vi "Test wrapper.vi"() -> ()   [LabVIEW 2009]
uses:
  <vilib>/Analysis/2dsp.llb/2D Complex FFT.vi
  <vilib>/Analysis/NI_AALPro.lvlib
panel:
  in  "Save\nAmplitudes":bool
  in  "deviceId":i32
  in  "Intensity":sgl[](array[numeric])=[1.0, 1.0, 1.0]
  in  "Polynomial Coefficients":sgl[](array[numeric])=[128.0, 0.0, 0.0, 40.0, 0.0, 0.0, 0.0, 0.0, 0.0, 0.0, 0.0, 0.0, 0.0, 0.0, 0.0, 0.0, 0.0, 0.0, 0.0, 0.0, 0.0, 0.0, 0.0, 0.0, 0.0, 0.0, 0.0, 0.0, 0.0, 0.0, 0.0, 0.0, 0.0, 0.0, 0.0, 0.0, 0.0, 0.0, 0.0, 0.0, 0.0, 0.0, 0.0, 0.0, 0.0, 0.0, 0.0, 0.0, 0.0, 0.0, 0.0, 0.0, 0.0, 0.0, 0.0, 0.0, 0.0, 0.0, 0.0, 0.0, 0.0, 0.0, 0.0, 0.0, 0.0, 0.0, 0.0, 0.0, 0.0, 0.0, 0.0, 0.0, 0.0, 0.0, 0.0, 0.0, 0.0, 0.0, 0.0, 0.0, 0.0, 0.0, 0.0, 0.0, 0.0, 0.0, 0.0, 0.0, 0.0, 0.0, 0.0, 0.0, 0.0, 0.0, 0.0, 0.0, 0.0, 0.0, 0.0, 0.0, 0.0, 0.0, 0.0, 0.0, 0.0, 0.0, 0.0, 0.0, 0.0, 0.0, 0.0, 0.0, 0.0, 0.0, 0.0, 0.0, 0.0, 0.0, 0.0, 0.0]
  in  "alpha RPC":sgl=1.0
  in  "Polynomial Order":i32=3 min=3 max=7 step=1
  in  "Use polynomial LUT":bool=TRUE
  out "error out":errorcluster
  in  "Aberration Correction On":bool
  in  "Aberration Correction":sgl[](array[numeric])=array[262144 elements]
  in  "TrueFrame":i32=3
  in  "Number of \ntime to execute":i32=1
  out "Average \nexecution time":dbl=nan
  in  "GO":bool
  in  "stop program":bool
  out "Amplitudes/weights":sgl[][](graph)=[[1.0001239, 1.0001477, 1.0001446, 1.0001416, 1.0001386, 1.0001358, 1.0001332, 1.0001305, 1.0001283, 1.0001258], [0.99984175, 0.99979293, 0.9997994, 0.99980545, 0.9998114, 0.9998169, 0.9998223, 0.99982744, 0.9998326, 0.9998372], [1.0000381, 1.0000628, 1.0000595, 1.0000563, 1.0000532, 1.0000505, 1.0000477, 1.0000453, 1.0000426, 1.0000404]]
  out "Calculated image plane":dbl[][](graph)
  out "Generated Hologram":u8[][](graph)
  in  "method":i32(ring)=1 items=["Lenses and Gratings (3D)", "Gerchberg-Saxton (3D)", "Gerchberg-Saxton FFT (2D)"]
  in  "z":sgl[](array[numeric])=[0.0, 0.0, 0.0]
  in  "y":sgl[](array[numeric])=[4.0, 5.0, -4.0]
  in  "x":sgl[](array[numeric])=[4.0, -4.0, 4.0]
  in  "N_iterations":i32=10
  in  "SLM enabled":bool
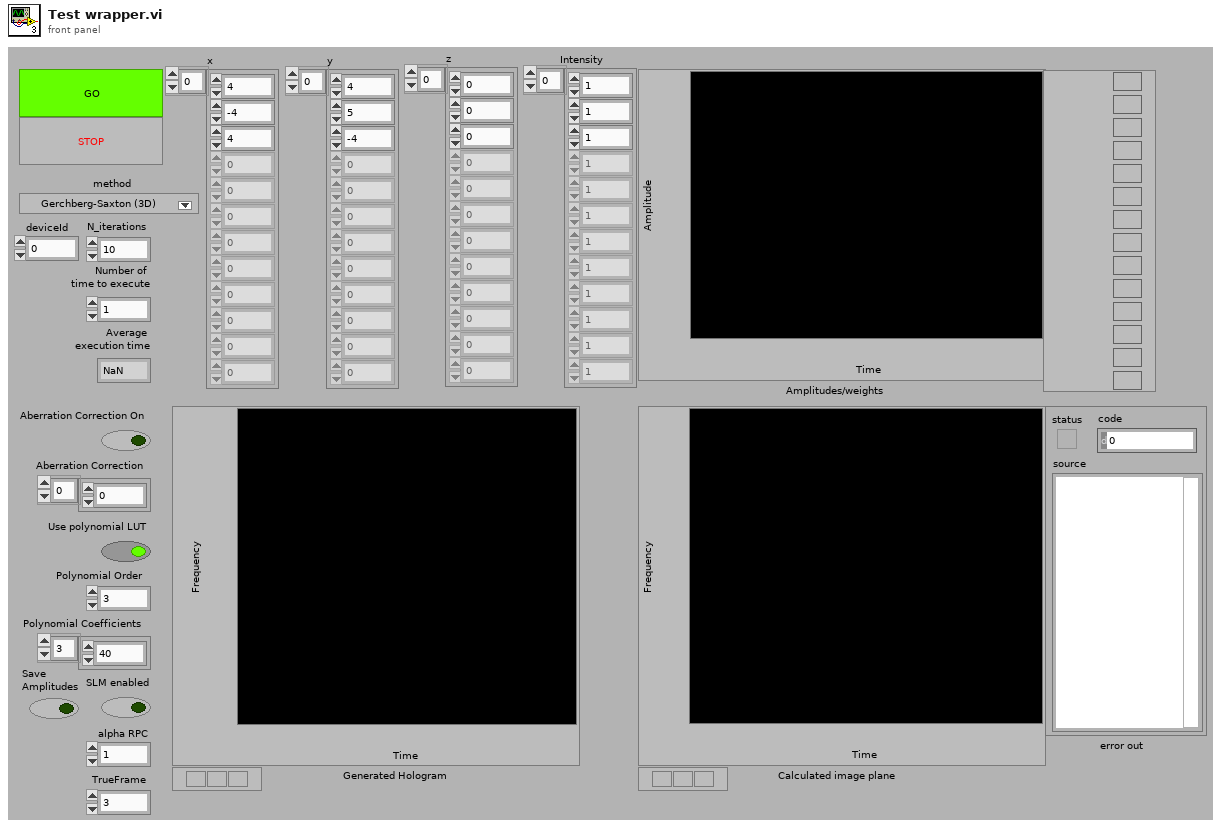
[diagram p1: front panel]
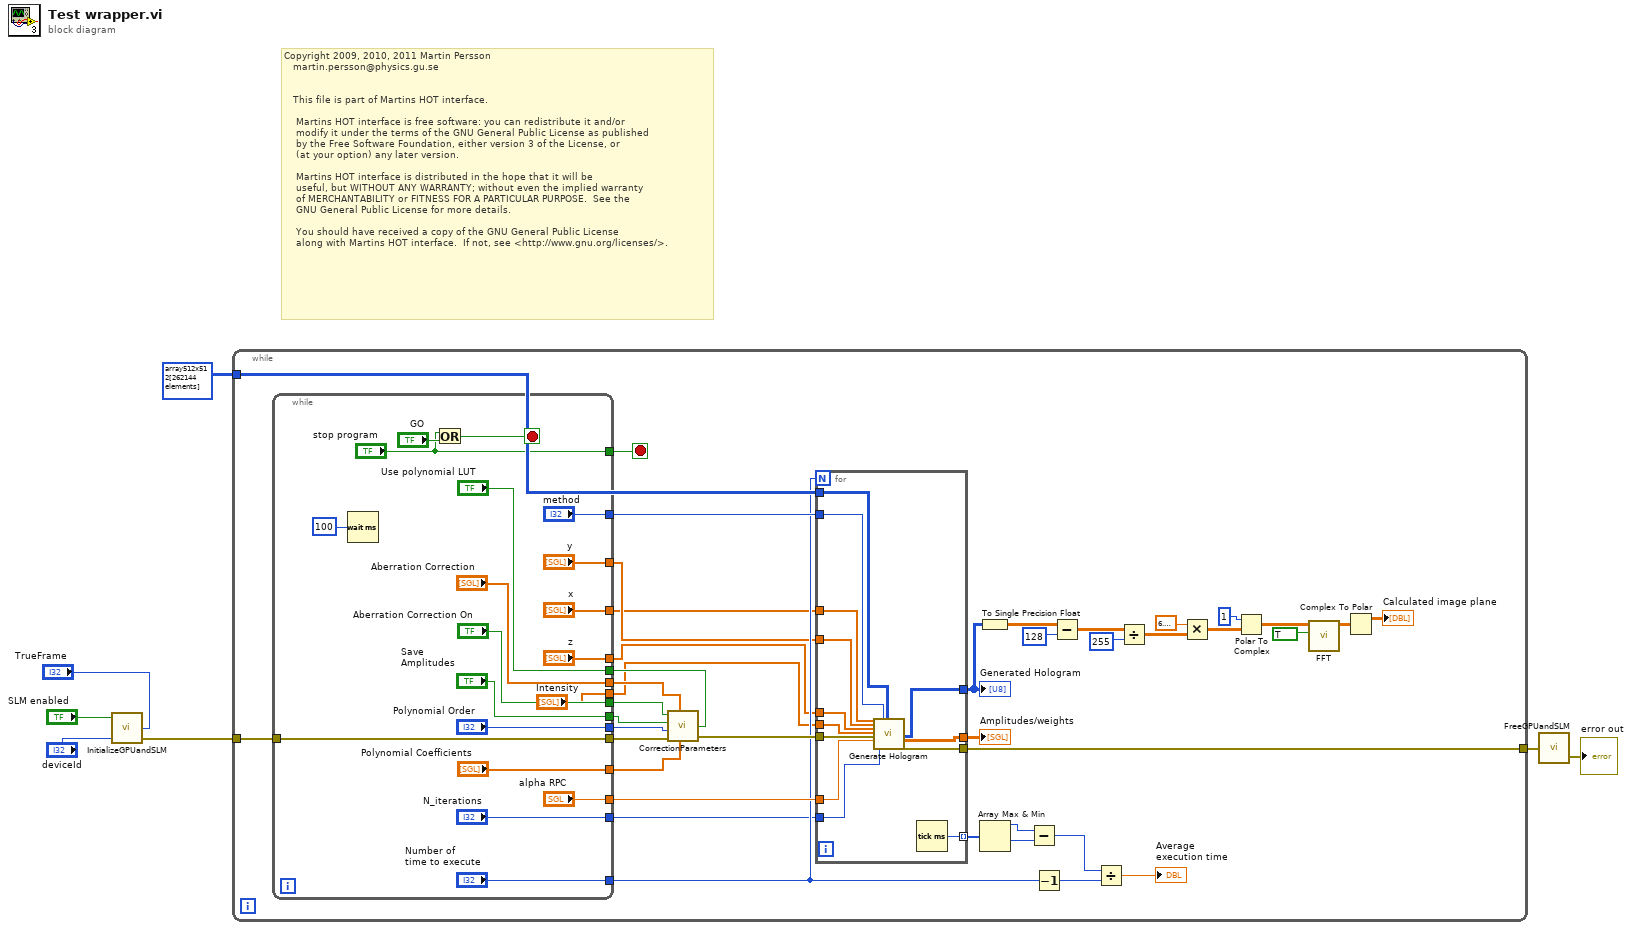
[diagram p0: block diagram]
diagram:
  # "Copyright 2009, 2010, 2011 Martin Persson \n   martin.persson@physics.gu.se\n\n\n   This file is part of Martins HOT interface.\n\n    Martins HOT interface is free software: you can redistribute it and/or \n    modify it under the terms of the GNU General Public License as published \n    by the Free Software Foundation, either version 3 of the License, or\n    (at your option) any later version.\n\n    Martins HOT interface is distributed in the hope that it will be \n    useful, but WITHOUT ANY WARRANTY; without even the implied warranty\n    of MERCHANTABILITY or FITNESS FOR A PARTICULAR PURPOSE.  See the\n    GNU General Public License for more details.\n\n    You should have received a copy of the GNU General Public License\n    along with Martins HOT interface.  If not, see <http://www.gnu.org/licenses/>."
  n1 = call "InitializeGPUandSLM.vi"("TrueFrame"="TrueFrame", "deviceId"="deviceId", "SLM enabled"="SLM enabled") -> ("CUDA/SLM error"=w1:errorcluster)  [unwired: 1 in, 1 out]
  n2 = while {
    tunnel: w1 -> [w24]
    tunnel: [w45] -> w6
    tunnel: u8[][] array512x512[262144 elements] ("Default") -> [w32]
    stop <- w46 stop-if-true
    n3 = while {
      tunnel: ["stop program"] -> w46
      tunnel: w24 -> [w75]
      tunnel: [w75] -> w23
      tunnel: ["alpha RPC"] -> w21
      tunnel: ["Use polynomial LUT"] -> w20
      tunnel: ["Aberration Correction On"] -> w19
      tunnel: ["method"] -> w18
      tunnel: ["Number of \ntime to execute"] -> w17
      tunnel: ["y"] -> w16
      tunnel: ["z"] -> w15
      tunnel: ["x"] -> w14
      tunnel: ["Polynomial Order"] -> w13
      tunnel: ["Aberration Correction"] -> w12
      tunnel: ["Polynomial Coefficients"] -> w11
      tunnel: ["N_iterations"] -> w10
      tunnel: ["Intensity"] -> w9
      tunnel: ["Save\nAmplitudes"] -> w8
      stop <- w77 stop-if-true
      n4 = Wait (ms)(milliseconds to wait=u32 100) -> ()  [unwired: 1 out]
      n5 = Or(x="stop program", y="GO") -> (x .or. y?=w77:bool)
    }
    n6 = call "CorrectionParameters.vi"("Aberration Correction On"=w19, "Aberration Correction"=w12, "SaveAmplitudes"=w8, "Polynomial Order"=w13, "Polynomial Coefficients"=w11, "error in"=w23, "Use polynomial LUT"=w20) -> ("error out"=w25:errorcluster)  [unwired: 1 out]
    n7 = for {
      N: w17 -> [_]
      tunnel: w25 -> [w60]
      tunnel: w10 -> [w59]
      tunnel: w16 -> [w58]
      tunnel: w15 -> [w57]
      tunnel: w18 -> [w56]
      tunnel: [w55] -> w47
      tunnel: [w54] -> w45
      tunnel: [w53] -> w33
      tunnel: w32 -> [w52]
      tunnel: w14 -> [w51]
      tunnel: w9 -> [w50]
      tunnel: [w49] -> w31 mode=indexing
      tunnel: w21 -> [w48]
      n8 = call "Generate Hologram.vi"("x"=w51, "y"=w58, "z"=w57, "spot_intensities"=w50, "CUDA/SLM error in"=w60, "alpha RPC"=w48, "N_iterations"=w59, "method"=w56, "CGH in"=w52) -> ("CGH out"=w53:u8[][], "weights"=w55:sgl[][], "CUDA/SLM error out"=w54:errorcluster)  [unwired: 16 in]
      n9 = Tick Count (ms)() -> (millisecond timer value=w49:u32)
    }
    "Generated Hologram" <- w33
    "Amplitudes/weights" <- w47
    n10 = To Single Precision Float(number=w33) -> (single precision float=w40:sgl[][])
    n11 = Array Max & Min(array=w31) -> (max value=w30:u32, min value=w29:u32)  [unwired: 2 out]
    n12 = Subtract(x=w30, y=w29) -> (x-y=w28:u32)
    n13 = Decrement(x=w17) -> (x-1=w22:i32)
    n14 = Subtract(x=w40, y=128) -> (x-y=w39:sgl[][])
    n15 = Divide(x=w28, y=w22) -> (x/y=→"Average \nexecution time":dbl)
    n16 = Divide(x=w39, y=255) -> (x/y=w42:sgl[][])
    n17 = Multiply(x=6.283185307179586, y=w42) -> (x*y=w36:dbl[][])
    n18 = Polar To Complex(1:w36, 2:1) -> (0:w35:cdb[][])
    n19 = call-poly <vilib>:"FFT.vi"("shift?"=TRUE, "X"=w35) -> ("FFT {X}"=w38:cdb[][])  [unwired: 2 in, 7 out]
    n20 = Complex To Polar(r * e^(i*theta)=w38) -> (r=→"Calculated image plane":dbl[][])  [unwired: 1 out]
  }
  n21 = call "FreeGPUandSLM.vi"("error in"=w6) -> ("error out"=→"error out":errorcluster)  [unwired: 1 out]
